vi "List.vi"(8 "error in (no error)":errorcluster) -> (0 "error out":errorcluster, 3 "registered loggers":string[](array[string]))   [LabVIEW 2018, in "GLog.lvlib" / "Registry.lvlib"]
uses:
  Registry.lvlib
  Registry Actions.ctl
  api/Utilities/Utilities.lvlib
panel:
  # "Connector Pane"
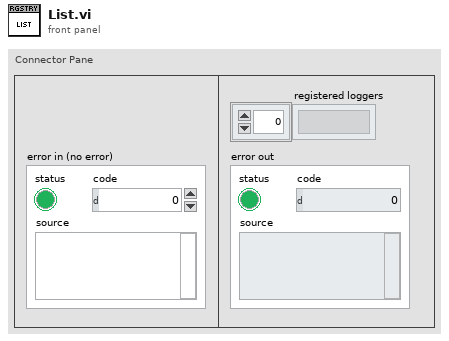
[diagram p1: front panel]
types:
  T1 = typedef "GLog.lvlib/Registry.lvlib/Registry Actions.ctl" = enum16{"Register", "Log", "Enable", "Enable All", "Disable", "Disable All", "List", "Unregister", "Unregister All"}
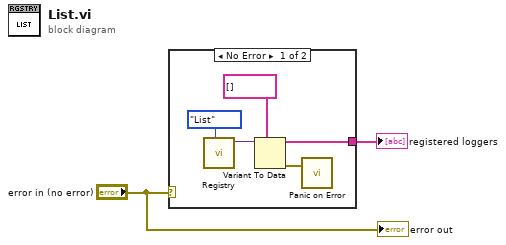
[diagram p0: block diagram]
diagram:
  n1 = case shown="No Error" "error in (no error)" {
    tunnel: [w4 _] -> w2
    frame No Error {
      n2 = call "Registry.vi"("action"=Registry_Actions."List") -> ("data out"=w6:variant)  [unwired: 9 in, 1 out]
      n3 = Variant To Data(type=string[] [], Variant=w6) -> (data=w4:string[], error out=w3:errorcluster)  [unwired: 1 in]
      n4 = call "Panic on Error.vi"("error in (no error)"=w3) -> ()  [unwired: 3 in]
    }
    frame Error {
    }
  }
  "registered loggers" <- w2
  "error out" <- "error in (no error)"
